vi "Certificate File Name.vi"(8 "error in (no error)":errorcluster caption="에러 입력(에러 없음)") -> (0 "error out":errorcluster caption="에러 출력", 2 "data sheet 파일명":string, 3 "성적서 파일명":string)   [LabVIEW 2020]
uses:
  Variables/Global_Cal Info.vi
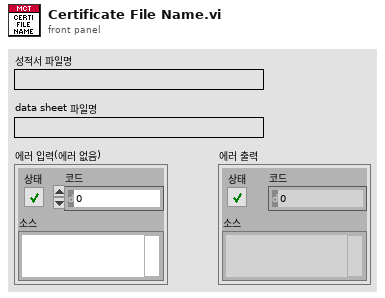
[diagram p1: front panel]
types:
  T1 = typedef "Clst_Cal Info Global.ctl" = cluster{"등록번호":string, "의뢰기관":string, "기기명":string, "제작회사":string, "형식":string, "기기번호":string, "소분류코드":string, "세부분류코드":string, "교정주기":string, "접수번호":string, "교정일자":string, "교정절차서 1":string, "교정절차서 2":string, "교정절차서 3":string, "접수확인자":string, "인증교정자":string, "기술책임자":string, "KOLAS 유무":string, "진행상태":string, "의뢰기관코드":string, "입고형태":string, "영문성적서?":bool, "합불판정?":bool, "부록?":bool, "절차서번호 1":string, "절차서번호 2":string, "절차서번호 3":string, "교정방식":string, "부서명":string}
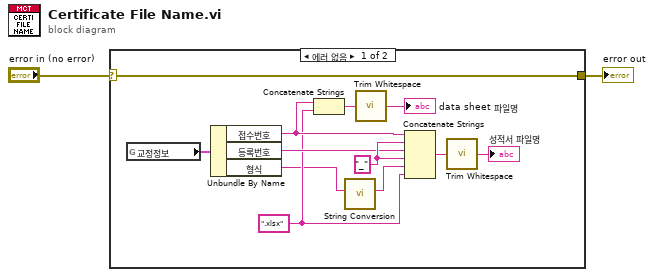
[diagram p0: block diagram]
diagram:
  n1 = case shown="에러 없음" "error in (no error)" {
    selector: "error in (no error)" -> [w11 w15]
    tunnel: [w11 w15] -> w2
    frame No Error {
      w8 = ".xlsx"
      w13 = "_"
      n2 = global read "Global_Cal Info.vi" "교정정보"() -> (w5:T1)
      n3 = Unbundle By Name(w5) -> ("접수번호"=w10:string, "등록번호"=w12:string, "형식"=w4:string)
      n4 = Concatenate Strings(w10, w8) -> (w9:string)
      n5 = call "String Conversion.vi"("문자열 입력"=w4) -> ("변경된 문자열 출력"=w3:string)  [unwired: 10 in]
      n6 = call <vilib>:"Trim Whitespace.vi"("string"=w9) -> ("trimmed string"=→"data sheet 파일명":string)  [unwired: 1 in]
      n7 = Concatenate Strings(w10, w13, w12, w13, w3, w8) -> (w14:string)
      n8 = call <vilib>:"Trim Whitespace.vi"("string"=w14) -> ("trimmed string"=→"성적서 파일명":string)  [unwired: 1 in]
    }
    frame Error {
    }
  }
  "error out" <- w2
